vi "Update Analysis Graph Poly.vi"   [LabVIEW 2023, in "Analysis Graph.lvclass"]
uses:
  Analysis Graph.lvclass
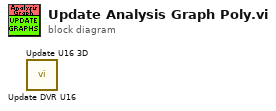
[diagram p0: block diagram]
diagram:
  n1 = call "Update DVR U16.vi"() -> ()  [unwired: 8 in, 4 out]
  n2 = call "Update U16 3D.vi"() -> ()  [unwired: 8 in, 4 out]
